vi "MAIN.vi"() -> ()   [LabVIEW 2016, in "副屏.lvlib"]
uses:
  <vilib>/Utility/miscctls.llb/LVPointTypeDef.ctl
  <vilib>/addons/database/_DB Variant To Data/Database Variant To Data.xnode
  PLC/PLC.lvlib
  <vilib>/Utility/config.llb/NI_LVConfig.lvlib
panel:
  out "单位":string
  out "测试浓度":string
  out "英文标题":string
  out "中文标题":string
  out "公司名称":string
  out "时间":string="2018"
  out "日":string="12"
  out "月":string="12"
  out "年":string="2018"
  # "年"
  # "月"
  # "日"
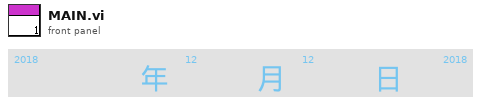
[diagram p1: front panel]
types:
  T1 = cluster{"显示参数中文名":string, "显示参数英文名":string, "显示浓度":string, "显示单位":string}
  T2 = typedef "LVPointTypeDef.ctl" = cluster{"Horizontal":i16, "Vertical":i16}
  T3 = typedef "NI_LVConfig.lvlib/Config Data RefNum.ctl" = refnum<k1>
  T4 = cluster{"AD0":sgl, "AD1":sgl, "AD2":sgl, "AD3":sgl, "AD4":sgl, "AD5":sgl}
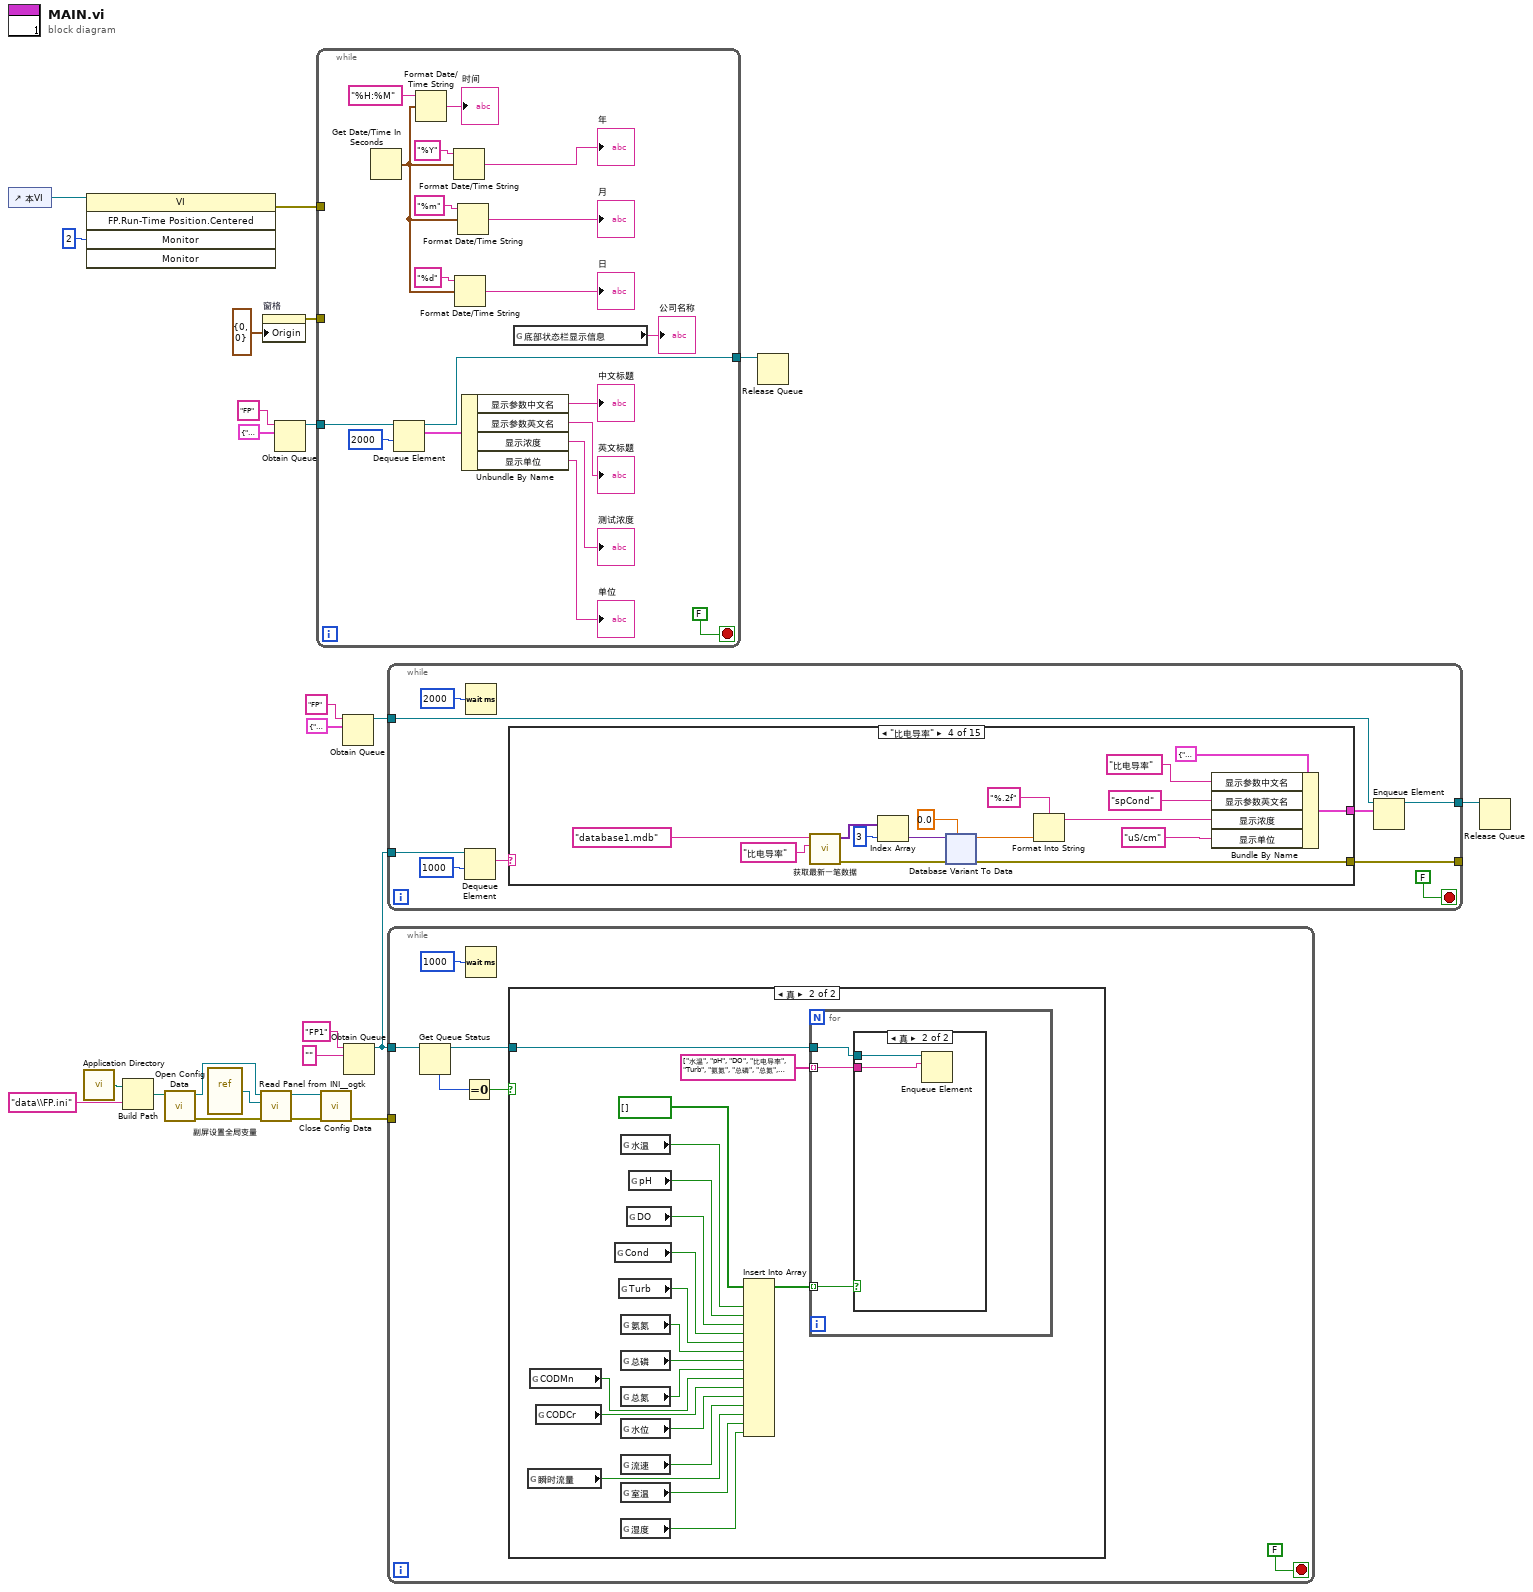
[diagram p0: block diagram]
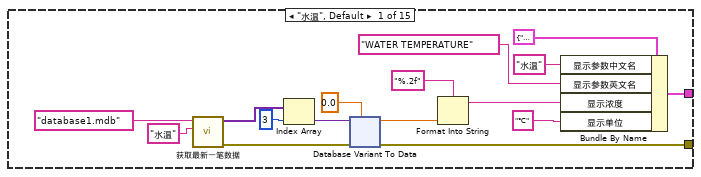
[diagram p4: hidden frame]
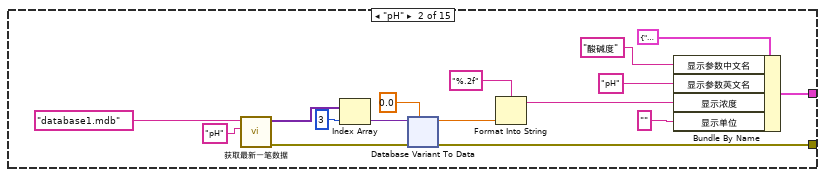
[diagram p5: hidden frame]
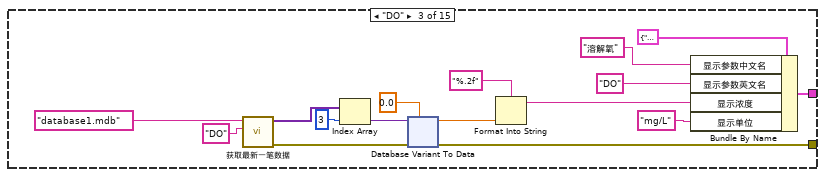
[diagram p6: hidden frame]
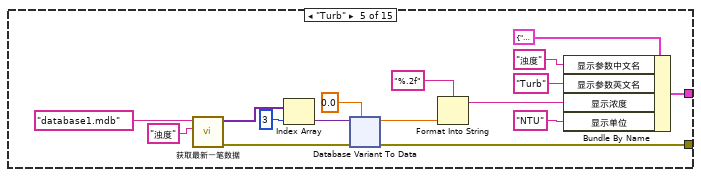
[diagram p7: hidden frame]
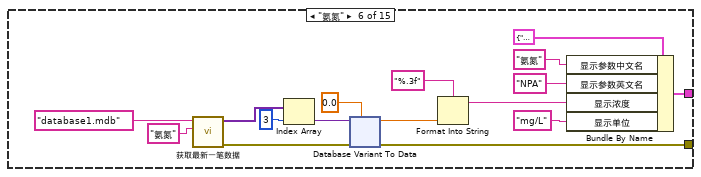
[diagram p8: hidden frame]
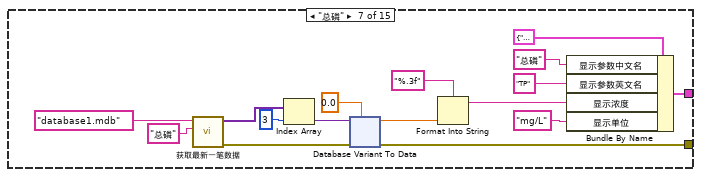
[diagram p9: hidden frame]
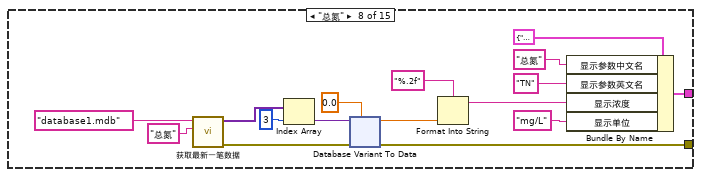
[diagram p10: hidden frame]
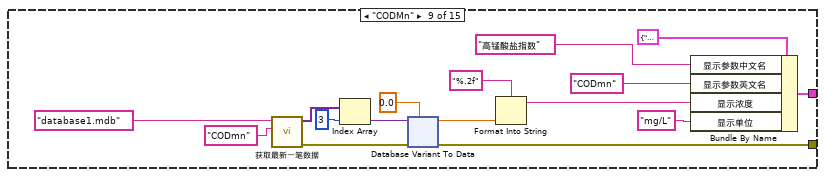
[diagram p11: hidden frame]
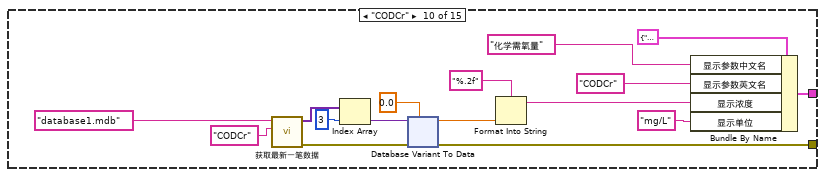
[diagram p12: hidden frame]
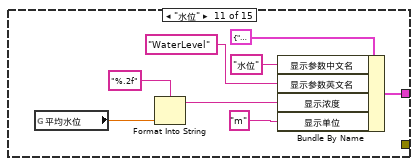
[diagram p13: hidden frame]
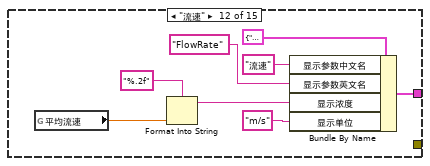
[diagram p14: hidden frame]
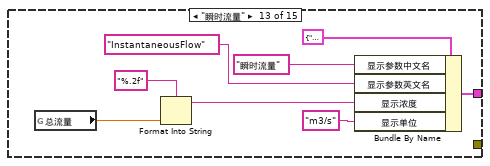
[diagram p15: hidden frame]
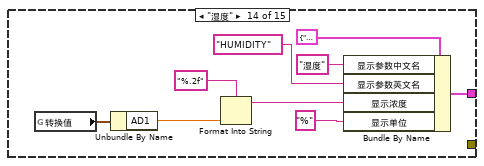
[diagram p16: hidden frame]
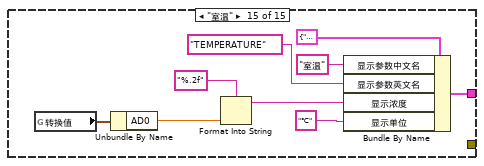
[diagram p17: hidden frame]
diagram:
  n1 = control-ref of="本VI"() -> (w3:refnum<vi>)
  n2 = call <vilib>:"Application Directory.vi"() -> ("Application Directory"=w12:path)
  n3 = invoke class="VI" method="FP.Run-Time Position.Centered"(reference=w3, "Monitor"=i16 2 ("显示器")) -> (error out=w1:errorcluster)  [unwired: 3 in, 4 out]
  n4 = Build Path(base path=w12, name or relative path="data\\FP.ini" ("名称或相对路径")) -> (appended path=w10:path)
  n5 = call <vilib>:"Open Config Data.vi"("configuration file path"=w10) -> ("error out"=w8:errorcluster, "refnum"=w5:T3)  [unwired: 8 in, 1 out]
  n6 = vi-ref "副屏设置全局变量.vi"() -> (w6:refnum<vi>)
  n7 = call <userlib>:"Read Panel from INI__ogtk.vi"("error in (no error)"=w8, "VI ref"=w6, "refnum"=w5) -> ("error out"=w7:errorcluster, "refnum out"=w4:T3)  [unwired: 7 in]
  n8 = property on="窗格" class="Pane"("Origin"=T2 {"Horizontal"=0, "Vertical"=0} ("原点")) -> (error out=w24:errorcluster)  [unwired: 2 in, 1 out]
  n9 = Obtain Queue(name (unnamed)="FP" ("名称（未命名）"), element data type=T1 {"显示参数中文名"="", "显示参数英文名"="", "显示浓度"="", "显示单位"=""}) -> (queue out=w21:refnum<queue>)  [unwired: 3 in, 2 out]
  n10 = while {
    tunnel: w24 -> [_]
    tunnel: w21 -> [w30]
    tunnel: [w28] -> w20
    tunnel: w1 -> [_]
    stop <- FALSE stop-if-true
    n11 = Get Date/Time In Seconds() -> (seconds since 1Jan1904=w36:timestamp)
    n12 = Dequeue Element(queue=w30, timeout in ms (-1)=2000 ("超时毫秒(-1)")) -> (queue out=w28:refnum<queue>, element=w29:T1)  [unwired: 1 in, 2 out]
    n13 = Format Date/Time String(time format string (%c)="%H:%M" ("时间格式字符串(%c)"), seconds (now)=w36) -> (date/time string=→"时间":string)  [unwired: 1 in]
    n14 = Format Date/Time String(time format string (%c)="%Y" ("时间格式字符串(%c)"), seconds (now)=w36) -> (date/time string=→"年":string)  [unwired: 1 in]
    n15 = Format Date/Time String(time format string (%c)="%d" ("时间格式字符串(%c)"), seconds (now)=w36) -> (date/time string=→"日":string)  [unwired: 1 in]
    n16 = Format Date/Time String(time format string (%c)="%m" ("时间格式字符串(%c)"), seconds (now)=w36) -> (date/time string=→"月":string)  [unwired: 1 in]
    n17 = Unbundle By Name(w29) -> ("显示参数中文名"=→"中文标题":string, "显示参数英文名"=→"英文标题":string, "显示浓度"=→"测试浓度":string, "显示单位"=→"单位":string)
    n18 = global read "副屏设置全局变量.vi" "底部状态栏显示信息"() -> (→"公司名称":string)
  }
  n19 = call <vilib>:"Close Config Data.vi"("error in (no error)"=w7, "refnum"=w4) -> ("error out"=w9:errorcluster)  [unwired: 8 in, 1 out]
  n20 = Obtain Queue(name (unnamed)="FP" ("名称（未命名）"), element data type=T1 {"显示参数中文名"="", "显示参数英文名"="", "显示浓度"="", "显示单位"=""}) -> (queue out=w17:refnum<queue>)  [unwired: 3 in, 2 out]
  n21 = Obtain Queue(name (unnamed)="FP1" ("名称（未命名）"), element data type="") -> (queue out=w13:refnum<queue>)  [unwired: 3 in, 2 out]
  n22 = while {
    tunnel: w17 -> [w53]
    tunnel: [w52] -> w16
    tunnel: [w48] -> _
    tunnel: w13 -> [w47]
    stop <- FALSE stop-if-true
    n23 = Dequeue Element(queue=w47, timeout in ms (-1)=1000 ("超时毫秒(-1)")) -> (element=w45:string)  [unwired: 1 in, 3 out]
    n24 = Wait (ms)(milliseconds to wait=u32 2000 ("等待时间（毫秒）")) -> ()  [unwired: 1 out]
    n25 = case shown="\"比电导率\"" w45 {
      tunnel: [w65 w113 w161 w209 w257 w305 w353 w401 w449 w497 w537 w545 w553 w562 w571] -> w49
      tunnel: [w54 w102 w150 w198 w246 w294 w342 w390 w438 w486 _ _ _ _ _] -> w48
      frame "水温", Default {
        n26 = call "获取最新一笔数据.vi"("table"="水温", "database"="database1.mdb" ("名称或相对路径")) -> ("error out"=w55:errorcluster, "子数组"=w61:variant[])  [unwired: 8 in]
        n27 = Index Array(array=w61, index=3 ("索引")) -> (element=w59:variant)
        n28 = xnode "Database Variant To Data"("database variant"=w59, "error in (no error)"=w55, "type"=0.0) -> ("data"=w56:dbl, "error out"=w54:errorcluster)
        n29 = Format Into String(format string="%.2f" ("格式字符串"), w56) -> (resulting string=w63:string)  [unwired: 2 in, 1 out]
        n30 = Bundle By Name(cluster=T1 {"显示参数中文名"="", "显示参数英文名"="", "显示浓度"="", "显示单位"=""} ("元素"), "显示参数中文名"="水温", "显示参数英文名"="WATER TEMPERATURE", "显示浓度"=w63, "显示单位"="℃") -> (w65:T1)
      }
      frame "pH" {
        n31 = call "获取最新一笔数据.vi"("table"="pH", "database"="database1.mdb" ("名称或相对路径")) -> ("error out"=w103:errorcluster, "子数组"=w109:variant[])  [unwired: 8 in]
        n32 = Index Array(array=w109, index=3 ("索引")) -> (element=w107:variant)
        n33 = xnode "Database Variant To Data"("database variant"=w107, "error in (no error)"=w103, "type"=0.0) -> ("data"=w104:dbl, "error out"=w102:errorcluster)
        n34 = Format Into String(format string="%.2f" ("格式字符串"), w104) -> (resulting string=w111:string)  [unwired: 2 in, 1 out]
        n35 = Bundle By Name(cluster=T1 {"显示参数中文名"="", "显示参数英文名"="", "显示浓度"="", "显示单位"=""} ("元素"), "显示参数中文名"="酸碱度", "显示参数英文名"="pH", "显示浓度"=w111, "显示单位"="") -> (w113:T1)
      }
      frame "DO" {
        n36 = call "获取最新一笔数据.vi"("table"="DO", "database"="database1.mdb" ("名称或相对路径")) -> ("error out"=w151:errorcluster, "子数组"=w157:variant[])  [unwired: 8 in]
        n37 = Index Array(array=w157, index=3 ("索引")) -> (element=w155:variant)
        n38 = xnode "Database Variant To Data"("database variant"=w155, "error in (no error)"=w151, "type"=0.0) -> ("data"=w152:dbl, "error out"=w150:errorcluster)
        n39 = Format Into String(format string="%.2f" ("格式字符串"), w152) -> (resulting string=w159:string)  [unwired: 2 in, 1 out]
        n40 = Bundle By Name(cluster=T1 {"显示参数中文名"="", "显示参数英文名"="", "显示浓度"="", "显示单位"=""} ("元素"), "显示参数中文名"="溶解氧", "显示参数英文名"="DO", "显示浓度"=w159, "显示单位"="mg/L") -> (w161:T1)
      }
      frame "比电导率" {
        n41 = call "获取最新一笔数据.vi"("table"="比电导率", "database"="database1.mdb" ("名称或相对路径")) -> ("error out"=w199:errorcluster, "子数组"=w205:variant[])  [unwired: 8 in]
        n42 = Index Array(array=w205, index=3 ("索引")) -> (element=w203:variant)
        n43 = xnode "Database Variant To Data"("database variant"=w203, "error in (no error)"=w199, "type"=0.0) -> ("data"=w200:dbl, "error out"=w198:errorcluster)
        n44 = Format Into String(format string="%.2f" ("格式字符串"), w200) -> (resulting string=w207:string)  [unwired: 2 in, 1 out]
        n45 = Bundle By Name(cluster=T1 {"显示参数中文名"="", "显示参数英文名"="", "显示浓度"="", "显示单位"=""} ("元素"), "显示参数中文名"="比电导率", "显示参数英文名"="spCond", "显示浓度"=w207, "显示单位"="uS/cm") -> (w209:T1)
      }
      frame "Turb" {
        n46 = call "获取最新一笔数据.vi"("table"="浊度", "database"="database1.mdb" ("名称或相对路径")) -> ("error out"=w247:errorcluster, "子数组"=w253:variant[])  [unwired: 8 in]
        n47 = Index Array(array=w253, index=3 ("索引")) -> (element=w251:variant)
        n48 = xnode "Database Variant To Data"("database variant"=w251, "error in (no error)"=w247, "type"=0.0) -> ("data"=w248:dbl, "error out"=w246:errorcluster)
        n49 = Format Into String(format string="%.2f" ("格式字符串"), w248) -> (resulting string=w255:string)  [unwired: 2 in, 1 out]
        n50 = Bundle By Name(cluster=T1 {"显示参数中文名"="", "显示参数英文名"="", "显示浓度"="", "显示单位"=""} ("元素"), "显示参数中文名"="浊度", "显示参数英文名"="Turb", "显示浓度"=w255, "显示单位"="NTU") -> (w257:T1)
      }
      frame "氨氮" {
        n51 = call "获取最新一笔数据.vi"("table"="氨氮", "database"="database1.mdb" ("名称或相对路径")) -> ("error out"=w295:errorcluster, "子数组"=w301:variant[])  [unwired: 8 in]
        n52 = Index Array(array=w301, index=3 ("索引")) -> (element=w299:variant)
        n53 = xnode "Database Variant To Data"("database variant"=w299, "error in (no error)"=w295, "type"=0.0) -> ("data"=w296:dbl, "error out"=w294:errorcluster)
        n54 = Format Into String(format string="%.3f" ("格式字符串"), w296) -> (resulting string=w303:string)  [unwired: 2 in, 1 out]
        n55 = Bundle By Name(cluster=T1 {"显示参数中文名"="", "显示参数英文名"="", "显示浓度"="", "显示单位"=""} ("元素"), "显示参数中文名"="氨氮", "显示参数英文名"="NPA", "显示浓度"=w303, "显示单位"="mg/L") -> (w305:T1)
      }
      frame "总磷" {
        n56 = call "获取最新一笔数据.vi"("table"="总磷", "database"="database1.mdb" ("名称或相对路径")) -> ("error out"=w343:errorcluster, "子数组"=w349:variant[])  [unwired: 8 in]
        n57 = Index Array(array=w349, index=3 ("索引")) -> (element=w347:variant)
        n58 = xnode "Database Variant To Data"("database variant"=w347, "error in (no error)"=w343, "type"=0.0) -> ("data"=w344:dbl, "error out"=w342:errorcluster)
        n59 = Format Into String(format string="%.3f" ("格式字符串"), w344) -> (resulting string=w351:string)  [unwired: 2 in, 1 out]
        n60 = Bundle By Name(cluster=T1 {"显示参数中文名"="", "显示参数英文名"="", "显示浓度"="", "显示单位"=""} ("元素"), "显示参数中文名"="总磷", "显示参数英文名"="TP", "显示浓度"=w351, "显示单位"="mg/L") -> (w353:T1)
      }
      frame "总氮" {
        n61 = call "获取最新一笔数据.vi"("table"="总氮", "database"="database1.mdb" ("名称或相对路径")) -> ("error out"=w391:errorcluster, "子数组"=w397:variant[])  [unwired: 8 in]
        n62 = Index Array(array=w397, index=3 ("索引")) -> (element=w395:variant)
        n63 = xnode "Database Variant To Data"("database variant"=w395, "error in (no error)"=w391, "type"=0.0) -> ("data"=w392:dbl, "error out"=w390:errorcluster)
        n64 = Format Into String(format string="%.2f" ("格式字符串"), w392) -> (resulting string=w399:string)  [unwired: 2 in, 1 out]
        n65 = Bundle By Name(cluster=T1 {"显示参数中文名"="", "显示参数英文名"="", "显示浓度"="", "显示单位"=""} ("元素"), "显示参数中文名"="总氮", "显示参数英文名"="TN", "显示浓度"=w399, "显示单位"="mg/L") -> (w401:T1)
      }
      frame "CODMn" {
        n66 = call "获取最新一笔数据.vi"("table"="CODmn", "database"="database1.mdb" ("名称或相对路径")) -> ("error out"=w439:errorcluster, "子数组"=w445:variant[])  [unwired: 8 in]
        n67 = Index Array(array=w445, index=3 ("索引")) -> (element=w443:variant)
        n68 = xnode "Database Variant To Data"("database variant"=w443, "error in (no error)"=w439, "type"=0.0) -> ("data"=w440:dbl, "error out"=w438:errorcluster)
        n69 = Format Into String(format string="%.2f" ("格式字符串"), w440) -> (resulting string=w447:string)  [unwired: 2 in, 1 out]
        n70 = Bundle By Name(cluster=T1 {"显示参数中文名"="", "显示参数英文名"="", "显示浓度"="", "显示单位"=""} ("元素"), "显示参数中文名"="高锰酸盐指数", "显示参数英文名"="CODmn", "显示浓度"=w447, "显示单位"="mg/L") -> (w449:T1)
      }
      frame "CODCr" {
        n71 = call "获取最新一笔数据.vi"("table"="CODCr", "database"="database1.mdb" ("名称或相对路径")) -> ("error out"=w487:errorcluster, "子数组"=w493:variant[])  [unwired: 8 in]
        n72 = Index Array(array=w493, index=3 ("索引")) -> (element=w491:variant)
        n73 = xnode "Database Variant To Data"("database variant"=w491, "error in (no error)"=w487, "type"=0.0) -> ("data"=w488:dbl, "error out"=w486:errorcluster)
        n74 = Format Into String(format string="%.2f" ("格式字符串"), w488) -> (resulting string=w495:string)  [unwired: 2 in, 1 out]
        n75 = Bundle By Name(cluster=T1 {"显示参数中文名"="", "显示参数英文名"="", "显示浓度"="", "显示单位"=""} ("元素"), "显示参数中文名"="化学需氧量", "显示参数英文名"="CODCr", "显示浓度"=w495, "显示单位"="mg/L") -> (w497:T1)
      }
      frame "水位" {
        n76 = global read "流量计全局变量.vi" "平均水位"() -> (w534:dbl)
        n77 = Format Into String(format string="%.2f" ("格式字符串"), w534) -> (resulting string=w535:string)  [unwired: 2 in, 1 out]
        n78 = Bundle By Name(cluster=T1 {"显示参数中文名"="", "显示参数英文名"="", "显示浓度"="", "显示单位"=""} ("元素"), "显示参数中文名"="水位", "显示参数英文名"="WaterLevel", "显示浓度"=w535, "显示单位"="m") -> (w537:T1)
      }
      frame "流速" {
        n79 = global read "流量计全局变量.vi" "平均流速"() -> (w542:dbl)
        n80 = Format Into String(format string="%.2f" ("格式字符串"), w542) -> (resulting string=w543:string)  [unwired: 2 in, 1 out]
        n81 = Bundle By Name(cluster=T1 {"显示参数中文名"="", "显示参数英文名"="", "显示浓度"="", "显示单位"=""} ("元素"), "显示参数中文名"="流速", "显示参数英文名"="FlowRate", "显示浓度"=w543, "显示单位"="m/s") -> (w545:T1)
      }
      frame "瞬时流量" {
        n82 = global read "流量计全局变量.vi" "总流量"() -> (w550:dbl)
        n83 = Format Into String(format string="%.2f" ("格式字符串"), w550) -> (resulting string=w551:string)  [unwired: 2 in, 1 out]
        n84 = Bundle By Name(cluster=T1 {"显示参数中文名"="", "显示参数英文名"="", "显示浓度"="", "显示单位"=""} ("元素"), "显示参数中文名"="瞬时流量", "显示参数英文名"="InstantaneousFlow", "显示浓度"=w551, "显示单位"="m3/s") -> (w553:T1)
      }
      frame "湿度" {
        n85 = global read "采配水全局变量.vi" "转换值"() -> (w559:T4)
        n86 = Unbundle By Name(w559) -> ("AD1"=w561:sgl)
        n87 = Format Into String(format string="%.2f" ("格式字符串"), w561) -> (resulting string=w558:string)  [unwired: 2 in, 1 out]
        n88 = Bundle By Name(cluster=T1 {"显示参数中文名"="", "显示参数英文名"="", "显示浓度"="", "显示单位"=""} ("元素"), "显示参数中文名"="湿度", "显示参数英文名"="HUMIDITY", "显示浓度"=w558, "显示单位"="%") -> (w562:T1)
      }
      frame "室温" {
        n89 = global read "采配水全局变量.vi" "转换值"() -> (w568:T4)
        n90 = Unbundle By Name(w568) -> ("AD0"=w570:sgl)
        n91 = Format Into String(format string="%.2f" ("格式字符串"), w570) -> (resulting string=w567:string)  [unwired: 2 in, 1 out]
        n92 = Bundle By Name(cluster=T1 {"显示参数中文名"="", "显示参数英文名"="", "显示浓度"="", "显示单位"=""} ("元素"), "显示参数中文名"="室温", "显示参数英文名"="TEMPERATURE", "显示浓度"=w567, "显示单位"="℃") -> (w571:T1)
      }
    }
    n93 = Enqueue Element(queue=w53, element=w49) -> (queue out=w52:refnum<queue>)  [unwired: 2 in, 2 out]
  }
  n94 = while {
    tunnel: w13 -> [w580]
    tunnel: w9 -> [_]
    stop <- FALSE stop-if-true
    n95 = Get Queue Status(queue=w580) -> (queue out=w577:refnum<queue>, # elements in queue=w579:i32)  [unwired: 2 in, 6 out]
    n96 = Equal To 0?(x=w579) -> (x = 0?=w578:bool)
    n97 = Wait (ms)(milliseconds to wait=u32 1000 ("等待时间（毫秒）")) -> ()  [unwired: 1 out]
    n98 = case shown="真" w578 {
      tunnel: w577 -> [_ w600]
      frame False {
      }
      frame True {
        n99 = global read "副屏设置全局变量.vi" "瞬时流量"() -> (w586:bool)
        n100 = global read "副屏设置全局变量.vi" "CODMn"() -> (w590:bool)
        n101 = global read "副屏设置全局变量.vi" "CODCr"() -> (w589:bool)
        n102 = global read "副屏设置全局变量.vi" "Cond"() -> (w595:bool)
        n103 = global read "副屏设置全局变量.vi" "Turb"() -> (w594:bool)
        n104 = global read "副屏设置全局变量.vi" "水温"() -> (w598:bool)
        n105 = global read "副屏设置全局变量.vi" "氨氮"() -> (w593:bool)
        n106 = global read "副屏设置全局变量.vi" "总磷"() -> (w592:bool)
        n107 = global read "副屏设置全局变量.vi" "总氮"() -> (w591:bool)
        n108 = global read "副屏设置全局变量.vi" "水位"() -> (w588:bool)
        n109 = global read "副屏设置全局变量.vi" "流速"() -> (w587:bool)
        n110 = global read "副屏设置全局变量.vi" "室温"() -> (w585:bool)
        n111 = global read "副屏设置全局变量.vi" "湿度"() -> (w584:bool)
        n112 = global read "副屏设置全局变量.vi" "DO"() -> (w596:bool)
        n113 = global read "副屏设置全局变量.vi" "pH"() -> (w597:bool)
        n114 = Insert Into Array(array=bool[] [], new element #1=w598, new element #2=w597, new element #3=w596, new element #4=w595, new element #5=w594, new element #6=w593, new element #7=w592, new element #8=w591, new element #9=w590, new element #10=w589, new element #11=w588, new element #12=w587, new element #13=w586, new element #14=w585, new element #15=w584) -> (w583:bool[])  [unwired: 1 in]
        n115 = for {
          tunnel: w600 -> [w603]
          tunnel: w583 -> [w602] mode=indexing
          tunnel: string[] ["水温", "pH", "DO", "比电导率", "Turb", "氨氮", "总磷", "总氮", "CODMn", "CODCr", "水位", "流速", "瞬时流量", "室温", "湿度"] -> [w601] mode=indexing
          n116 = case shown="真" w602 {
            tunnel: w603 -> [_ w605]
            tunnel: w601 -> [_ w604]
            frame False {
            }
            frame True {
              n117 = Enqueue Element(queue=w605, element=w604) -> ()  [unwired: 2 in, 3 out]
            }
          }
        }
      }
    }
  }
  n118 = Release Queue(queue=w20) -> ()  [unwired: 2 in, 3 out]
  n119 = Release Queue(queue=w16) -> ()  [unwired: 2 in, 3 out]
